vi "Write Values.vi"(8 "error in (no error)":errorcluster, 10 "Buses":refnum<class "Abs_Type.lvclass">[](array[class]), 11 "Bus_Access in":refnum<class "Bus_Access.lvclass">) -> (0 "error out":errorcluster, 3 "Bus_Access out":refnum<class "Bus_Access.lvclass">)   [LabVIEW 2021, in "Bus_Access.lvclass"]
uses:
  Bus_Access.lvclass
  <vilib>/TSA/Abstract Data Classes/Abs_Types/Type/Abs_Type.lvclass
  Bus_Access.lvclass/Bus_Access.ctl
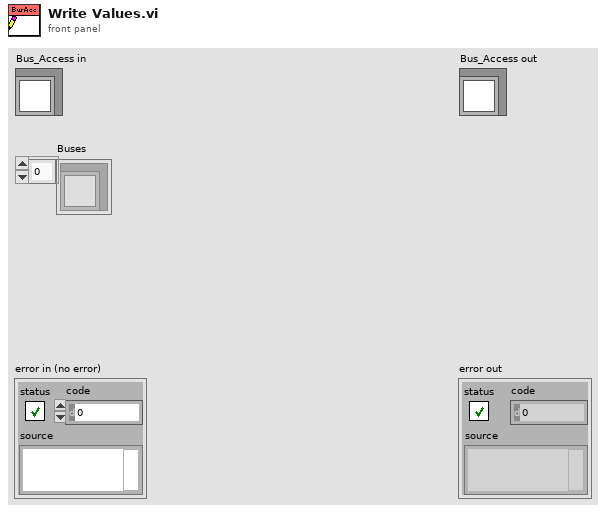
[diagram p1: front panel]
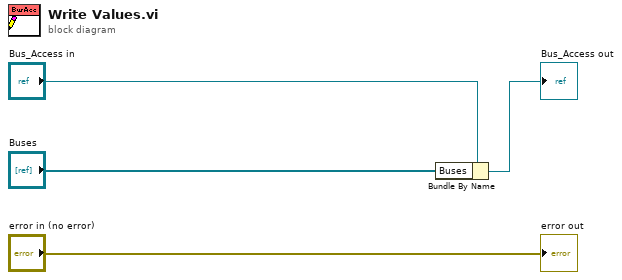
[diagram p0: block diagram]
diagram:
  n1 = Bundle By Name(cluster="Bus_Access in", "Buses"="Buses") -> (→"Bus_Access out":refnum<class "Bus_Access.lvclass">)
  "error out" <- "error in (no error)"
